vi "AlliGator Reorder Decay Pre-processing Operations.vi"(8 "Error In":errorcluster, 11 "Ring in":refnum<vi>) -> (0 "Error Out":errorcluster)   [LabVIEW 2021, in "AlliGator Settings.lvlib"]
doc: "Dialog window allowing the user to reorder decay pre-processing steps."
uses:
  AlliGator Settings.lvlib
  Arrays/Array Element Reordering.ctl
  06c9731b-b29d-433c-b3f3-a398076bdc61.vi
  93a8a00b-629f-42c8-bc34-743edd25a182.vi
  58554703-94c4-417d-b25e-666c14c86f3d.vi
  abebfc73-200f-48f5-9880-bfb49c2a3f24.vi
  Arrays/Arrays.lvlib
panel:
  in  "OK Button":bool caption="OK"
  in  "Cancel Button":bool caption="Cancel"
  in  "Bottom Button":bool caption="Bottom"
  in  "Top Button":bool caption="Top"
  in  "Down Button":bool caption="Down"
  in  "Up Button":bool caption="Up"
  in  "Decay Preprocessing Operations Order":i32(listbox)
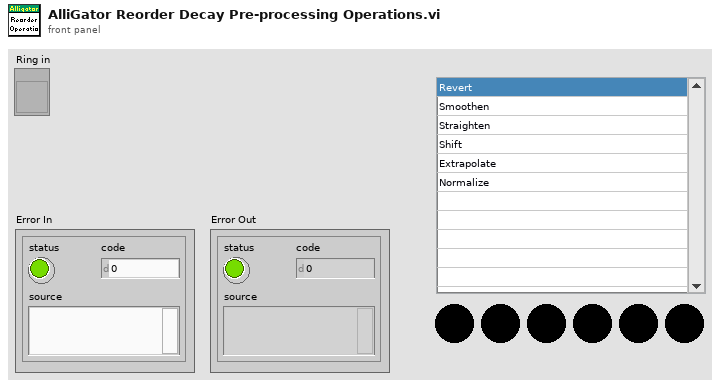
[diagram p1: front panel]
types:
  T1 = typedef "Arrays.lvlib/Array Element Reordering.ctl" = enum16{"top", "up", "down", "bottom"}
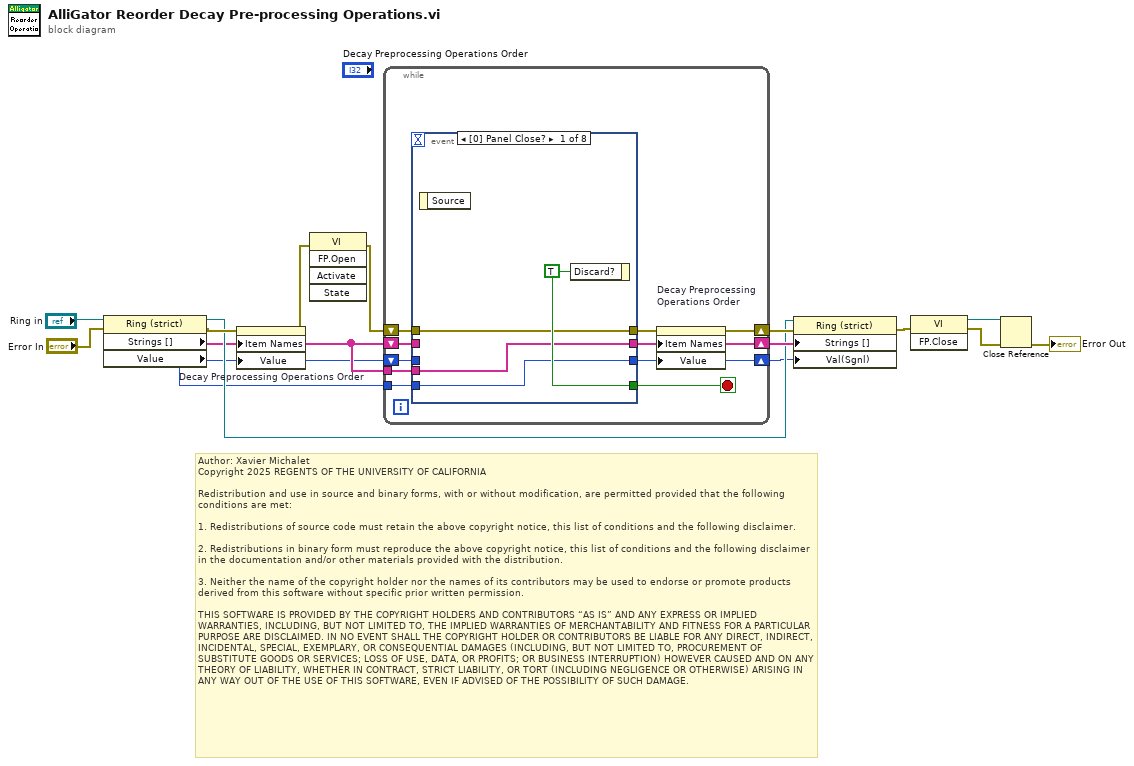
[diagram p0: block diagram]
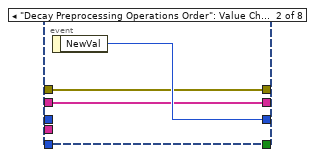
[diagram p2: hidden frame]
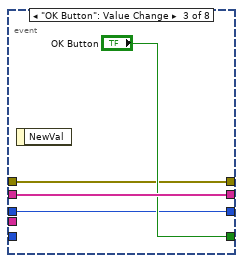
[diagram p3: hidden frame]
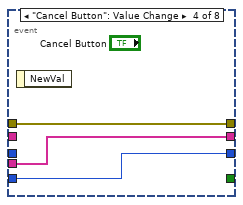
[diagram p4: hidden frame]
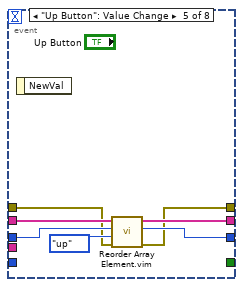
[diagram p5: hidden frame]
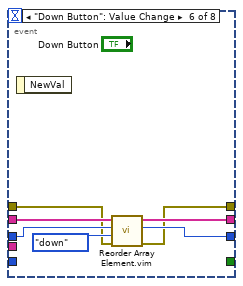
[diagram p6: hidden frame]
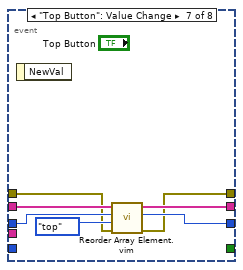
[diagram p7: hidden frame]
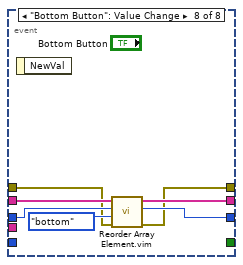
[diagram p8: hidden frame]
diagram:
  # "Author: Xavier Michalet\nCopyright 2025 REGENTS OF THE UNIVERSITY OF CALIFORNIA\n\nRedistribution and use in source and binary forms, with or without modification, are permitted provided that the following conditions are met:\n\n1. Redistributions of source code must retain the above copyright notice, this list of conditions and the following disclaimer.\n\n2. Redistributions in binary form must reproduce the above copyright notice, this list of conditions and the following disclaimer in the documentation and/or other materials provided with the distribution.\n\n3. Neither the name of the copyright holder nor the names of its contributors may be used to endorse or promote products derived from this software without specific prior written permission.\n\nTHIS SOFTWARE IS PROVIDED BY THE COPYRIGHT HOLDERS AND CONTRIBUTORS “AS IS” AND ANY EXPRESS OR IMPLIED WARRANTIES, INCLUDING, BUT NOT LIMITED TO, THE IMPLIED WARRANTIES OF MERCHANTABILITY AND FITNESS FOR A PARTICULAR PURPOSE ARE DISCLAIMED. IN NO EVENT SHALL THE COPYRIGHT HOLDER OR CONTRIBUTORS BE LIABLE FOR ANY DIRECT, INDIRECT, INCIDENTAL, SPECIAL, EXEMPLARY, OR CONSEQUENTIAL DAMAGES (INCLUDING, BUT NOT LIMITED TO, PROCUREMENT OF SUBSTITUTE GOODS OR SERVICES; LOSS OF USE, DATA, OR PROFITS; OR BUSINESS INTERRUPTION) HOWEVER CAUSED AND ON ANY THEORY OF LIABILITY, WHETHER IN CONTRACT, STRICT LIABILITY, OR TORT (INCLUDING NEGLIGENCE OR OTHERWISE) ARISING IN ANY WAY OUT OF THE USE OF THIS SOFTWARE, EVEN IF ADVISED OF THE POSSIBILITY OF SUCH DAMAGE."
  n1 = property class="Ring (strict)"(reference="Ring in", error in="Error In") -> (reference out=w10:refnum<vi>, error out=w14:errorcluster, "Strings []"=w9:string[], "Value"=w2:u16)
  n2 = property on="Decay Preprocessing Operations Order" class="LstBox (strict)"(error in=w14, "Item Names"=w9, "Value"=w2) -> (error out=w4:errorcluster)  [unwired: 1 in, 1 out]
  n3 = invoke class="VI" method="FP.Open"(error in=w4) -> (error out=w3:errorcluster)  [unwired: 4 in, 4 out]
  n4 = while {
    shift-right: [w21] -> w12
    shift-left: w3 -> [w23]
    shift-right: [w19] -> w11
    shift-left: w9 -> [w24]
    tunnel: w9 -> [w20]
    tunnel: w2 -> [w18]
    shift-right: [w16] -> w1
    shift-left: w2 -> [w17]
    stop <- w25 stop-if-true
    n5 = event shown="[0] Panel Close?" {
      selector: _ -> [_ _ _ _ _ _ _ _]
      dyn-events: _ -> [_ _ _ _ _ _ _ _]
      timeout: _ -> [_ _ _ _ _ _ _ _]
      tunnel: [w29 _ "OK Button" _ _ _ _ _] -> w25
      tunnel: w24 -> [_ w30 w36 _ w45 w52 w59 w66]
      tunnel: w17 -> [_ _ w33 _ w44 w51 w58 w65]
      tunnel: [w27 w30 w36 w39 w46 w53 w60 w67] -> w19
      tunnel: [w26 w32 w33 w37 w42 w49 w56 w63] -> w16
      tunnel: w23 -> [w28 w31 w34 w38 w41 w48 w55 w62]
      tunnel: [w28 w31 w34 w38 w40 w47 w54 w61] -> w22
      tunnel: w20 -> [w27 _ _ w39 _ _ _ _]
      tunnel: w18 -> [w26 _ _ w37 _ _ _ _]
      event Panel Close? {
        w29 = TRUE ("Discard?")
        n6 = event-data() -> ()  [unwired: 1 in, 1 out]
        n7 = event-data("Discard?"=w29) -> ()  [unwired: 1 in, 1 out]
      }
      event "Decay Preprocessing Operations Order": Value Change {
        n8 = event-data() -> ("NewVal"=w32:i32)  [unwired: 1 in]
      }
      event "OK Button": Value Change {
        n9 = event-data() -> ()  [unwired: 1 in, 1 out]
      }
      event "Cancel Button": Value Change {
        n10 = event-data() -> ()  [unwired: 1 in, 1 out]
      }
      event "Up Button": Value Change {
        n11 = event-data() -> ()  [unwired: 1 in, 1 out]
        n12 = call "Reorder Array Element.vim"("Error In"=w41, "Operation"=Array_Element_Reordering."up", "index in"=w44, "Array in"=w45) -> ("Error Out"=w40:errorcluster, "index out"=w42:i32, "Array out"=w46:string[])  [unwired: 5 in]
      }
      event "Down Button": Value Change {
        n13 = event-data() -> ()  [unwired: 1 in, 1 out]
        n14 = call "Reorder Array Element.vim"("Error In"=w48, "Operation"=Array_Element_Reordering."down", "index in"=w51, "Array in"=w52) -> ("Error Out"=w47:errorcluster, "index out"=w49:i32, "Array out"=w53:string[])  [unwired: 5 in]
      }
      event "Top Button": Value Change {
        n15 = event-data() -> ()  [unwired: 1 in, 1 out]
        n16 = call "Reorder Array Element.vim"("Error In"=w55, "Operation"=Array_Element_Reordering."top", "index in"=w58, "Array in"=w59) -> ("Error Out"=w54:errorcluster, "index out"=w56:i32, "Array out"=w60:string[])  [unwired: 5 in]
      }
      event "Bottom Button": Value Change {
        n17 = event-data() -> ()  [unwired: 1 in, 1 out]
        n18 = call "Reorder Array Element.vim"("Error In"=w62, "Operation"=Array_Element_Reordering."bottom", "index in"=w65, "Array in"=w66) -> ("Error Out"=w61:errorcluster, "index out"=w63:i32, "Array out"=w67:string[])  [unwired: 5 in]
      }
    }
    n19 = property on="Decay Preprocessing Operations Order" class="LstBox (strict)"(error in=w22, "Item Names"=w19, "Value"=w16) -> (error out=w21:errorcluster)  [unwired: 1 in, 1 out]
  }
  n20 = property class="Ring (strict)"(reference=w10, error in=w12, "Strings []"=w11, "Val(Sgnl)"=w1) -> (error out=w8:errorcluster)  [unwired: 1 out]
  n21 = invoke class="VI" method="FP.Close"(error in=w8) -> (reference out=w7:refnum<vi>, error out=w6:errorcluster)  [unwired: 2 in, 1 out]
  n22 = Close Reference(reference=w7, error in (no error)=w6) -> (error out=→"Error Out":errorcluster)
